vi "Generate Sequence.vi"(8 "error in (no error)":errorcluster, 11 "WS5100 in":refnum<class "WS5100.lvclass">) -> (0 "error out":errorcluster, 3 "WS5100 out":refnum<class "WS5100.lvclass">)   [LabVIEW 2020, in "WS5100.lvclass"]
uses:
  WS5100.lvclass
  C:/Sandbox/Git_Sandbox/WiSpry Test Framework source code (LV20)/WiSpry Test Framework/Devices/NI DAQmx/NI DAQmx.lvclass
  C:/Sandbox/Git_Sandbox/WiSpry Test Framework source code (LV20)/WiSpry Test Framework/Devices/Device.lvclass
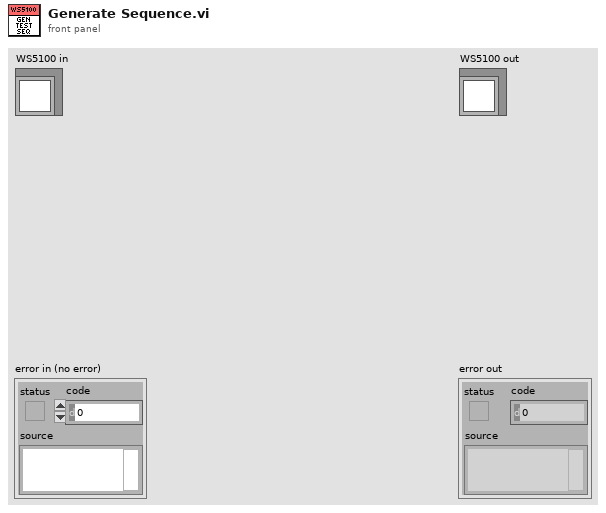
[diagram p1: front panel]
types:
  T1 = cluster{"GPIO Settings":bool[][], "GPIO Values":string[]}
  T2 = enum16{"Vdd", "Control 0", "Control 1", "Control 2", "Control 3"}[]
  T3 = typedef "NI DAQmx.lvclass/DAQmx line name.ctl" = cluster{"lines":tag, "Function":string, "Function":enum16{"Vdd", "Control 0", "Control 1", "Control 2", "Control 3"}}
  T4 = enum16{"Vdd", "Control 0", "Control 1", "Control 2", "Control 3"}
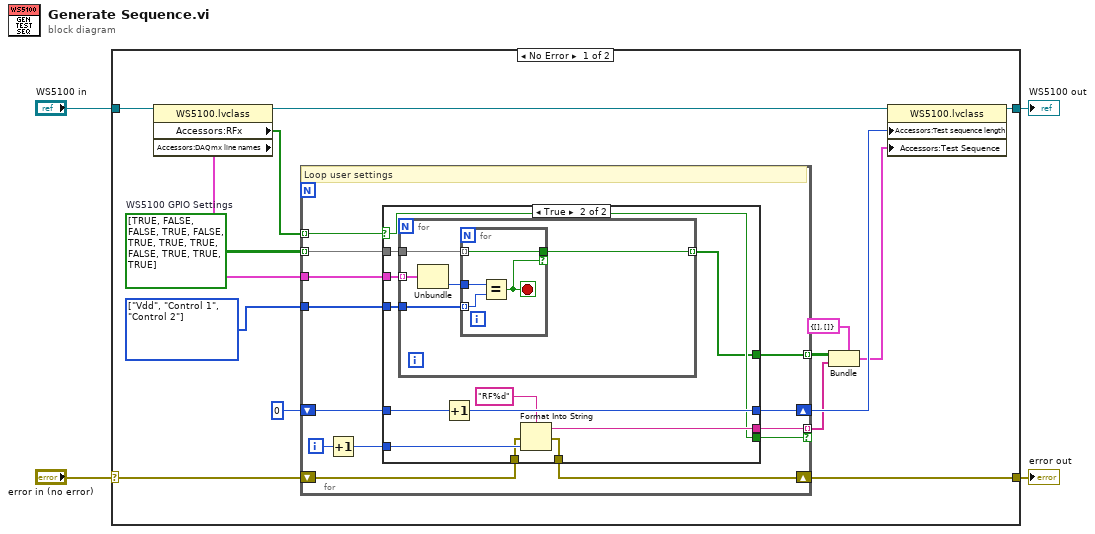
[diagram p0: block diagram]
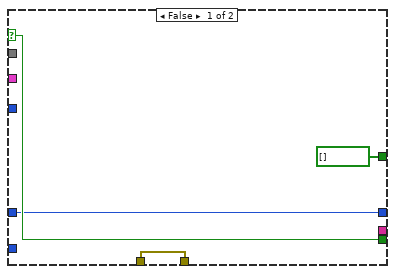
[diagram p2: hidden frame]
diagram:
  n1 = case shown="No Error" "error in (no error)" {
    selector: "error in (no error)" -> [w6 w59]
    tunnel: [w5 w59] -> w3
    tunnel: [w11 w58] -> w1
    tunnel: "WS5100 in" -> [w19 w58]
    frame No Error {
      w15 = T2 [enum."Vdd", enum."Control 1", enum."Control 2"] items=["Vdd", "Control 0", "Control 1", "Control 2", "Control 3"]
      w16 = bool[][] [[TRUE, FALSE, FALSE], [TRUE, FALSE, TRUE], [TRUE, TRUE, FALSE], [TRUE, TRUE, TRUE]]  # WS5100 GPIO Settings
      n2 = property class="WS5100.lvclass"(reference=w19) -> (reference out=w12:refnum<class "WS5100.lvclass">, "Accessors:RFx"=w18:bool[], "Accessors:DAQmx line names"=w17:T3[])  [unwired: 1 in, 1 out]
      n3 = for {
        tunnel: w18 -> [w28] mode=indexing
        tunnel: w17 -> [w31]
        tunnel: w16 -> [w29] mode=indexing
        tunnel: w15 -> [w30]
        shift-right: [w26] -> w13
        shift-left: 0 -> [w27]
        tunnel: [w24] -> w10 mode=indexing if=w23
        tunnel: [w22] -> w9 mode=indexing
        shift-right: [w20] -> w5
        shift-left: w6 -> [w21]
        i -> [w32]
        # "Loop user settings"
        n4 = Increment(x=w32) -> (x+1=w25:i32)
        n5 = case shown="True" w28 {
          selector: w28 -> [w36 w40]
          tunnel: w31 -> [_ w48]
          tunnel: w30 -> [_ w47]
          tunnel: w29 -> [_ w46]
          tunnel: w27 -> [w35 w45]
          tunnel: [w35 w44] -> w26
          tunnel: w25 -> [_ w42]
          tunnel: [_ w41] -> w24
          tunnel: [w36 w40] -> w23
          tunnel: [bool[] [] w39] -> w22
          tunnel: w21 -> [w33 w38]
          tunnel: [w33 w37] -> w20
          frame False {
          }
          frame True {
            n6 = for {
              tunnel: w48 -> [w53] mode=indexing
              tunnel: w47 -> [w52]
              tunnel: w46 -> [w50]
              tunnel: [w49] -> w39 mode=indexing
              n7 = Unbundle(w53) -> ("Function"=w51:T4)  [unwired: 2 out]
              n8 = for {
                tunnel: w52 -> [w56] mode=indexing
                tunnel: w51 -> [w57]
                tunnel: w50 -> [w55] mode=indexing
                tunnel: [w55] -> w49 if=w54
                stop <- w54 stop-if-true
                n9 = Equal?(x=w57, y=w56) -> (x = y?=w54:bool)
              }
            }
            n10 = Increment(x=w45) -> (x+1=w44:i32)
            n11 = Format Into String(format string="RF%d", error in=w38, w42) -> (resulting string=w41:string, error out=w37:errorcluster)  [unwired: 1 in]
          }
        }
      }
      n12 = Bundle(cluster=T1 {"GPIO Settings"=[], "GPIO Values"=[]} ("Test Sequence"), "GPIO Settings"=w9, "GPIO Values"=w10) -> (w7:T1)
      n13 = property class="WS5100.lvclass"(reference=w12, "Accessors:Test sequence length"=w13, "Accessors:Test Sequence"=w7) -> (reference out=w11:refnum<class "WS5100.lvclass">)  [unwired: 1 in, 1 out]
    }
    frame Error {
    }
  }
  "error out" <- w3
  "WS5100 out" <- w1
